vi "reenable verification.vi"(8 "error in":errorcluster, 11 "config in":u64) -> (0 "error out":errorcluster)   [LabVIEW 2016, in "lv tls dll.lvlib"]
uses:
  lv tls dll.lvlib
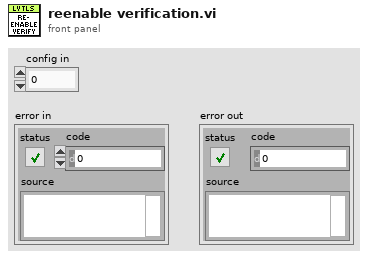
[diagram p1: front panel]
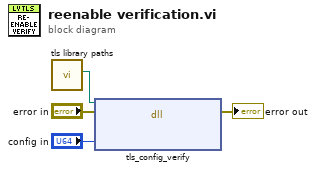
[diagram p0: block diagram]
diagram:
  n1 = call "tls library paths.vi"() -> ("libtls"=w1:path)  [unwired: 10 in, 1 out]
  n2 = dll-call lib="C:/Users/IEUser/Desktop/tlssimple/libtls-15.dll" fn="tls_config_verify"(path in=w1, error in="error in", "config"="config in") -> (error out=→"error out":errorcluster)  [unwired: 3 in, 1 out]
